vi "đọc biển số xe.vi"() -> ()   [LabVIEW 2020]
uses:
  <vilib>/userdefined/High Color/IMAQdx.ctl
  <vilib>/vision/driver/NI_Vision_Acquisition_Software.lvlib
  <vilib>/vision/NI_Vision_Development_Module.lvlib
panel:
  out "result":string
  in  "Rectangle":T1 {"Rotation" min=-90.0 max=90.0 step=1.0 format="%.2f"; "Left" scale=0.0..1024.0; "Right" scale=0.0..1024.0}
  in  "File Path":path
  out "Image":T2(plugin-control)
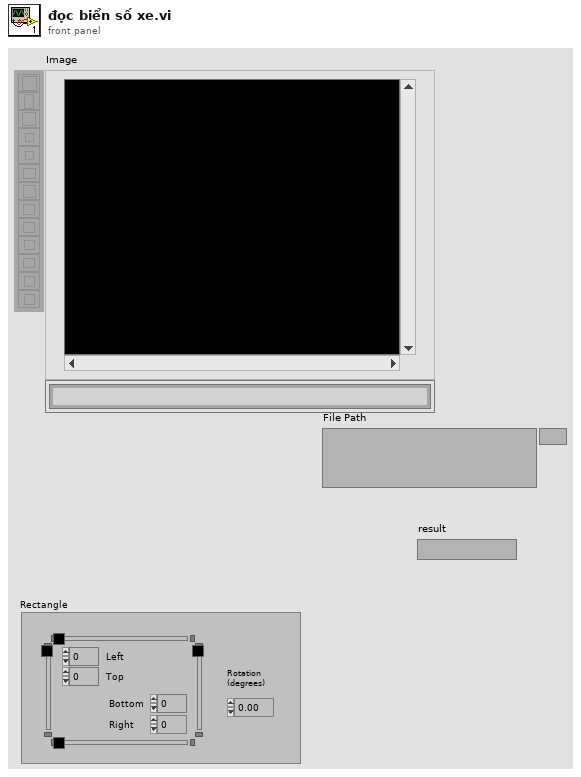
[diagram p1: front panel]
types:
  T1 = typedef "IMAQ Rectangle" = cluster{"Left":i32, "Top":i32, "Right":i32, "Bottom":i32, "Rotation":dbl}
  T2 = typedef "IMAQ Image.ctl" = refnum<image>
  T3 = typedef "IMAQdx.ctl" = refnum<k21>
  T4 = typedef "IMAQ OCR Session.ctl" = refnum<k1>
  T5 = typedef "ROI Descriptor" = cluster{"Global Rectangle":i32[], "Contours":cluster{"ID":enum32{"External", "Internal"}, "Type":u32, "Coordinates":i32[]}[]}
  T6 = cluster{"Global Rectangle":i32[], "Contours":cluster{"ID":enum32{"External", "Internal"}, "Type":u32, "Coordinates":i32[]}[]}
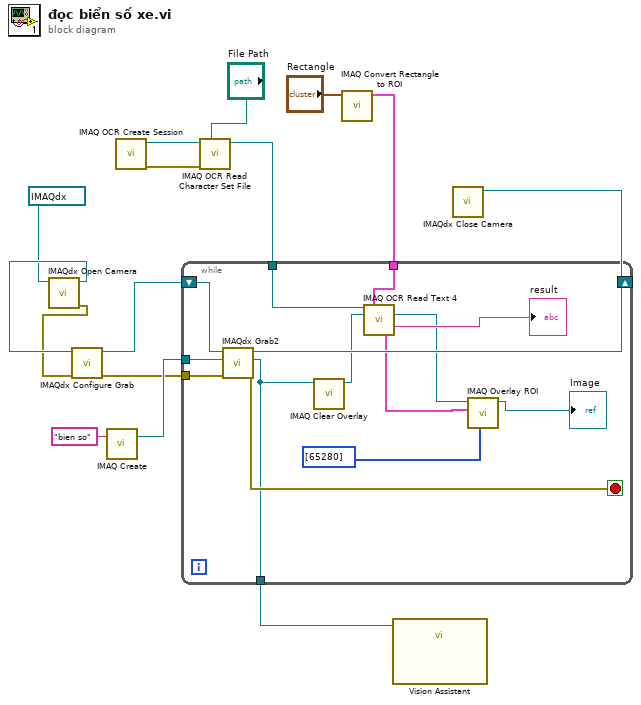
[diagram p0: block diagram]
diagram:
  n1 = call <vilib>:"IMAQdx Open Camera.vi"("Session In"=T3 "cam0") -> ("error out"=w1:errorcluster, "Session Out"=w15:T3)  [unwired: 9 in]
  n2 = call <vilib>:"IMAQdx Configure Grab.vi"("error in"=w1, "Session In"=w15) -> ("error out"=w10:errorcluster, "Session Out"=w14:T3)  [unwired: 8 in]
  n3 = call "IMAQ Create"("Image Name"="bien so") -> ("New Image"=w13:T2)  [unwired: 4 in, 1 out]
  n4 = call "IMAQ OCR Create Session"() -> ("error out"=w6:errorcluster, "IMAQ OCR Session"=w7:T4)  [unwired: 10 in]
  n5 = call "IMAQ OCR Read Character Set File"("File Path"="File Path", "error in (no error)"=w6, "IMAQ OCR Session"=w7) -> ("IMAQ OCR Session (dup)"=w5:T4)  [unwired: 6 in, 2 out]
  n6 = call "IMAQ Convert Rectangle to ROI"("Rectangle"="Rectangle") -> ("ROI Descriptor"=w3:T5)  [unwired: 8 in, 1 out]
  n7 = while {
    tunnel: w13 -> [w28]
    tunnel: w10 -> [w26]
    shift-right: [w27] -> w11
    shift-left: w14 -> [w29]
    tunnel: w5 -> [w25]
    tunnel: w3 -> [w24]
    tunnel: [w18] -> w2
    stop <- w22 stop-if-true
    n8 = call <vilib>:"IMAQdx Grab2.vi"("error in"=w26, "Image In"=w28, "Session In"=w29) -> ("error out"=w22:errorcluster, "Image Out"=w18:T2, "Session Out"=w27:T3)  [unwired: 5 in, 1 out]
    n9 = call "IMAQ Clear Overlay"("Image"=w18) -> ("Image Out"=w16:T2)  [unwired: 9 in, 1 out]
    n10 = call "IMAQ OCR Read Text 4"("IMAQ OCR Session"=w25, "ROI Descriptor"=w24, "Image"=w16) -> ("Image (dup)"=w17:T2, "Read String"=→"result":string, "ROI Bounding Characters"=w21:T6)  [unwired: 6 in, 4 out]
    n11 = call "IMAQ Overlay ROI"("Colors (Green)"=u32[] [65280], "ROI Descriptor"=w21, "Image"=w17) -> ("Image Out"=→"Image":T2)  [unwired: 7 in, 1 out]
  }
  n12 = call "Vision Assistant"("Image In"=w2) -> ()  [unwired: 25 in, 2 out]
  n13 = call <vilib>:"IMAQdx Close Camera.vi"("Session In"=w11) -> ()  [unwired: 10 in, 1 out]
